vi "cRIO_4DOF_Jacobian_v3.vi"(6 "XD":cdb, 9 "YD":cdb, 10 "ZD":cdb, 11 "Joint positions":dbl[](array[numeric])) -> (2 "J":dbl[][](array[numeric]))   [LabVIEW 2019]
uses:
  Global 1.vi
  <vilib>/imath/engines/lvmath2/RunTimeEngine/RowToken/NIMS_RowToken_CV_CV.vi
  <instcachedir>/0/NIMS_RowToken_CV_CV_63F97581FD6E4B12A13161F912ED327E.lvgen/NIMS_RowToken_CV_CV_63F97581FD6E4B12A13161F912ED327E_001.vi
  <vilib>/imath/engines/lvmath2/RunTimeEngine/RowToken/NIMS_RowToken_M_CV.vi
  <instcachedir>/0/NIMS_RowToken_M_CV_9FCC62D0D76A4B3BA956B702DD83EF32.lvgen/NIMS_RowToken_M_CV_9FCC62D0D76A4B3BA956B702DD83EF32_001.vi
  <vilib>/imath/engines/lvmath2/RunTimeEngine/ErrorHandling/NIMS_Create Error From Enums.vi
  <vilib>/imath/engines/lvmath2/RunTimeEngine/BuiltInFunctions/cross/NIMS_cross(GV,GV).vi
  <instcachedir>/0/NIMS_cross(GV,GV)_6F1F1C643EFF41C8A983D972A94A5A15.lvgen/NIMS_cross(GV,GV)_6F1F1C643EFF41C8A983D972A94A5A15_000.vi
  <vilib>/imath/engines/lvmath2/RunTimeEngine/ArithmeticOperatorToken/NIMS_ArithmeticOperator_multmx(RV,CV).vi
  <instcachedir>/0/NIMS_ArithmeticOperator_multmx(RV,CV)_029D7144B0004D0C96337D0595167468.lvgen/NIMS_ArithmeticOperator_multmx(RV,CV)_029D7144B0004D0C96337D0595167468_001.vi
  <vilib>/imath/engines/lvmath2/RunTimeEngine/RowToken/NIMS_RowToken_M_M.vi
  <instcachedir>/0/NIMS_RowToken_M_M_21FE36D058524603B8B587AC30FD72C2.lvgen/NIMS_RowToken_M_M_21FE36D058524603B8B587AC30FD72C2_003.vi
  <vilib>/imath/engines/lvmath2/RunTimeEngine/BuiltInFunctions/diag/NIMS_diag.vi
  <instcachedir>/0/NIMS_diag_DCAB8C8FDAF64F9E84492BB524435AA9.lvgen/NIMS_diag_DCAB8C8FDAF64F9E84492BB524435AA9_002.vi
  <vilib>/imath/engines/lvmath2/RunTimeEngine/BuiltInFunctions/inv/NIMS_inv(GM).vi
  <instcachedir>/0/NIMS_inv(GM)_A6DF8FE880224208AACFE4CF9F659502.lvgen/NIMS_inv(GM)_A6DF8FE880224208AACFE4CF9F659502_001.vi
  <vilib>/imath/engines/lvmath2/RunTimeEngine/ArithmeticOperatorToken/NIMS_ArithmeticOperator_multmx.vi
  <instcachedir>/0/NIMS_ArithmeticOperator_multmx_77F1D2D6F4D94BA7A97C4E7185C02392.lvgen/NIMS_ArithmeticOperator_multmx_77F1D2D6F4D94BA7A97C4E7185C02392_003.vi
  <vilib>/imath/engines/lvmath2/RunTimeEngine/IndexReplace/NIMS M(R2,R2)=M.vi
  <instcachedir>/0/NIMS M(R2,R2)=M_2398776730AD4DFB8507FC940586F47D.lvgen/NIMS M(R2,R2)=M_2398776730AD4DFB8507FC940586F47D_001.vi
  <vilib>/imath/engines/lvmath2/RunTimeEngine/IndexReplace/NIMS M(S,S)=S.vi
  <instcachedir>/0/NIMS M(S,S)=S_F60428D0350A4667AE68E0C0372F4DD1.lvgen/NIMS M(S,S)=S_F60428D0350A4667AE68E0C0372F4DD1_001.vi
  <vilib>/imathl/engines/lvmath/Functions/Error Handling/Create Error.vi
  <vilib>/imath/engines/lvmath2/RunTimeEngine/NodeEndStatement/NIMS_NodeEndStatement_Output.vi
  <instcachedir>/0/NIMS_NodeEndStatement_Output_53EC0D466D134D7ABD903AC30B43404B.lvgen/NIMS_NodeEndStatement_Output_53EC0D466D134D7ABD903AC30B43404B_000.vi
  <instcachedir>/0/NIMS_NodeEndStatement_Output_53EC0D466D134D7ABD903AC30B43404B.lvgen/NIMS_NodeEndStatement_Output_53EC0D466D134D7ABD903AC30B43404B_005.vi
  <instcachedir>/0/NIMS_NodeEndStatement_Output_53EC0D466D134D7ABD903AC30B43404B.lvgen/NIMS_NodeEndStatement_Output_53EC0D466D134D7ABD903AC30B43404B_002.vi
  <vilib>/imath/engines/lvmath2/RunTimeEngine/ErrorHandling/NIMS_Finalize Error.vi
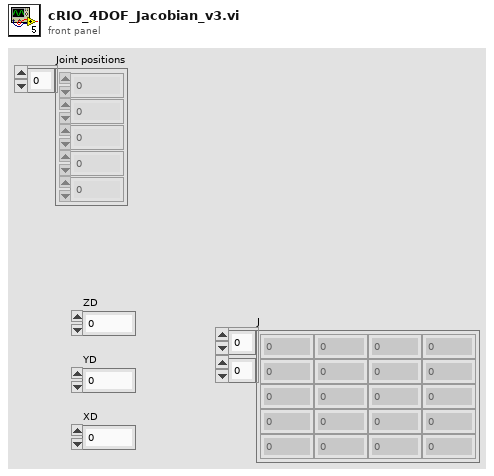
[diagram p1: front panel]
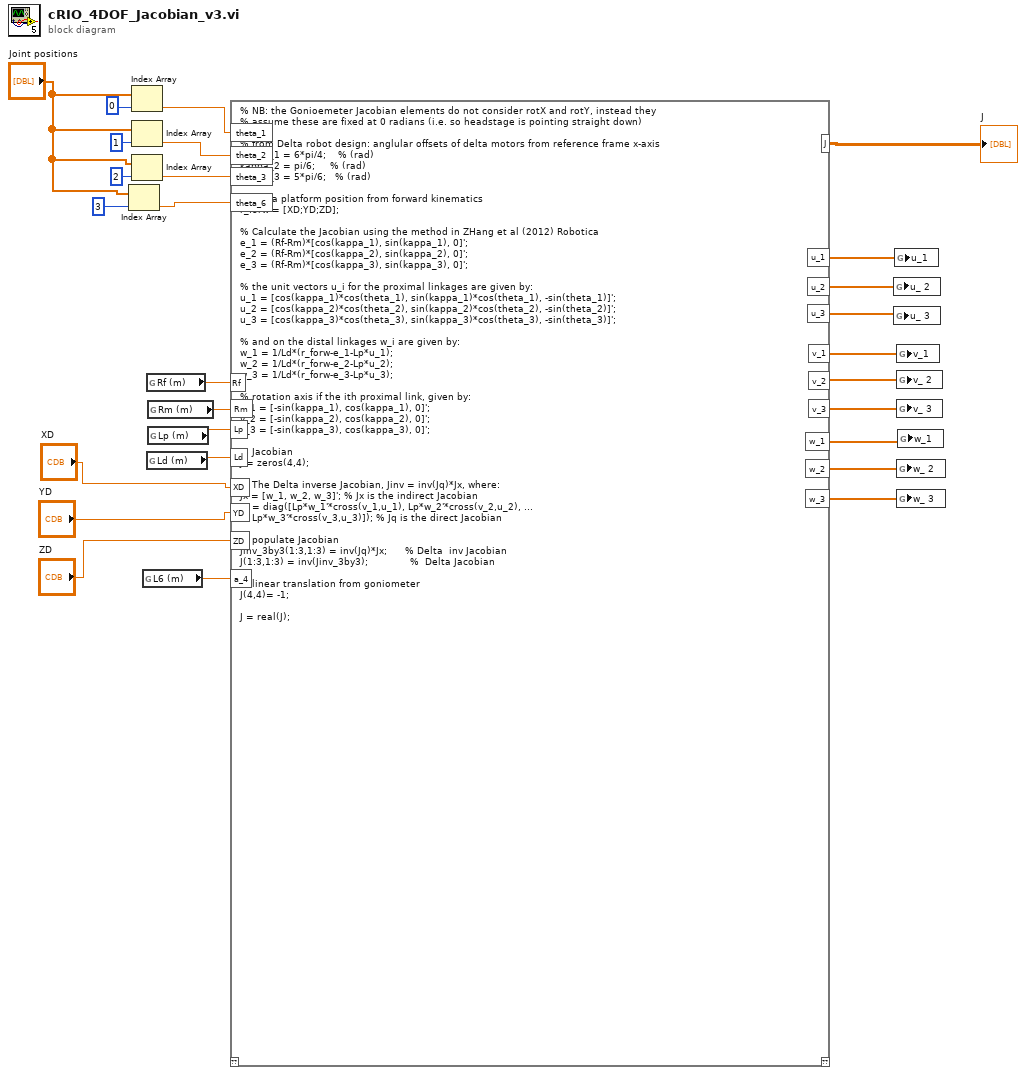
[diagram p0: block diagram]
diagram:
  n1 = Index Array(array="Joint positions", index=3) -> (element=w24:dbl)
  n2 = Index Array(array="Joint positions", index=0) -> (element=w21:dbl)
  n3 = Index Array(array="Joint positions", index=1) -> (element=w22:dbl)
  n4 = Index Array(array="Joint positions", index=2) -> (element=w23:dbl)
  n5 = global read "Global 1.vi" "L6 (m)"() -> (w10:dbl)
  n6 = global read "Global 1.vi" "Rf (m)"() -> (w14:dbl)
  n7 = global read "Global 1.vi" "Ld (m)"() -> (w11:dbl)
  n8 = global read "Global 1.vi" "Rm (m)"() -> (w13:dbl)
  n9 = global read "Global 1.vi" "Lp (m)"() -> (w12:dbl)
  n10 = mathscript code="% NB: the Gonioemeter Jacobian elements do not consider rotX and rotY, instead they \n% assume these are fixed at 0 radians (i.e. so headstage is pointing straight down)\n\n% from Delta robot design: anglular offsets of delta motors from reference frame x-axis\nkappa_1 = 6*pi/4;    % (rad)\nkappa_2 = pi/6;     % (rad)\nkappa_3 = 5*pi/6;   % (rad)\n\n% Delta platform position from forward kinematics\nr_forw = [XD;YD;ZD];\n\n% Calculate the Jacobian using the method in ZHang et al (2012) Robotica\ne_1 = (Rf-Rm)*[cos(kappa_1), sin(kappa_1), 0]';\ne_2 = (Rf-Rm)*[cos(kappa_2), sin(kappa_2), 0]';\ne_3 = (Rf-Rm)*[cos(kappa_3), sin(kappa_3), 0]';\n\n% the unit vectors u_i for the proximal linkages are given by: \nu_1 = [cos(kappa_1)*cos(theta_1), sin(kappa_1)*cos(theta_1), -sin(theta_1)]';\nu_2 = [cos(kappa_2)*cos(theta_2), sin(kappa_2)*cos(theta_2), -sin(theta_2)]';\nu_3 = [cos(kappa_3)*cos(theta_3), sin(kappa_3)*cos(theta_3), -sin(theta_3)]';\n\n% and on the distal linkages w_i are given by:\nw_1 = 1/Ld*(r_forw-e_1-Lp*u_1);\nw_2 = 1/Ld*(r_forw-e_2-Lp*u_2);\nw_3 = 1/Ld*(r_forw-e_3-Lp*u_3);\n\n% rotation axis if the ith proximal link, given by:\nv_1 = [-sin(kappa_1), cos(kappa_1), 0]';\nv_2 = [-sin(kappa_2), cos(kappa_2), 0]';\nv_3 = [-sin(kappa_3), cos(kappa_3), 0]';\n\n% Jacobian\nJ = zeros(4,4);\n\n% The Delta inverse Jacobian, Jinv = inv(Jq)*Jx, where: \nJx = [w_1, w_2, w_3]'; % Jx is the indirect Jacobian\nJq = diag([Lp*w_1'*cross(v_1,u_1), Lp*w_2'*cross(v_2,u_2), ...\n    Lp*w_3'*cross(v_3,u_3)]); % Jq is the direct Jacobian\n\n% populate Jacobian\nJinv_3by3(1:3,1:3) = inv(Jq)*Jx;      % Delta  inv Jacobian\nJ(1:3,1:3) = inv(Jinv_3by3);              %  Delta Jacobian\n\n% linear translation from goniometer\nJ(4,4)= -1;\n\nJ = real(J);"("theta_1"=w21, "theta_2"=w22, "theta_3"=w23, "Rf"=w14, "Rm"=w13, "Ld"=w11, "Lp"=w12, "XD"="XD", "YD"="YD", "ZD"="ZD", "theta_6"=w24, "a_4"=w10) -> ("J"=→"J":dbl[][], "u_1"=w9:dbl[], "u_2"=w8:dbl[], "u_3"=w7:dbl[], "v_1"=w6:dbl[], "v_2"=w5:dbl[], "v_3"=w4:dbl[], "w_1"=w3:cdb[], "w_2"=w2:cdb[], "w_3"=w1:cdb[])  [unwired: 1 in, 1 out]
  n11 = global write "Global 1.vi" "u_ 2"(w8) -> ()
  n12 = global write "Global 1.vi" "u_ 3"(w7) -> ()
  n13 = global write "Global 1.vi" "u_1"(w9) -> ()
  n14 = global write "Global 1.vi" "v_1"(w6) -> ()
  n15 = global write "Global 1.vi" "v_ 2"(w5) -> ()
  n16 = global write "Global 1.vi" "v_ 3"(w4) -> ()
  n17 = global write "Global 1.vi" "w_ 2"(w2) -> ()
  n18 = global write "Global 1.vi" "w_ 3"(w1) -> ()
  n19 = global write "Global 1.vi" "w_1"(w3) -> ()
